vi "NotchCoeffSingleChanQTemplate.vi"(0 "notch frequency":dbl=2.0 format="%#_6p", 5 "Q factor":dbl=20.0 format="%#_6p", 9 "sample rate":dbl=50000.0 format="%#_6p", 11 "error in (no error)":errorcluster) -> (4 "scaled coefficients":i32[](array[numeric]), 15 "error out":errorcluster)   [LabVIEW 2017, in "NI_FpgaMspHost.lvlib"]
doc: "This VI designs a Butterworth filter, then quantizes and formats the coefficients into 32-bit integers for use by the Butterworth Filter VI on the FPGA.\n\nThe user is responsible for ensuring that the configuration is valid. The following restrictions apply:\nCutoff frequency must meet Nyquist criterion.\nMultichannel filters are restricted to 2nd order.\nFilter order and type cannot be changed at run-time."
uses:
  <vilib>/rvi/Analysis/host/Public/NI_FpgaMspHost.lvlib
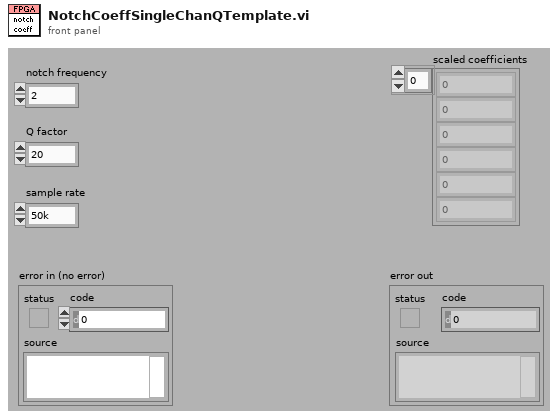
[diagram p1: front panel]
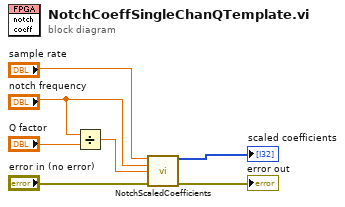
[diagram p0: block diagram]
diagram:
  n1 = Divide(x="notch frequency", y="Q factor") -> (x/y=w1:dbl)
  n2 = call <vilib>:"NotchScaledCoefficients.vi"("sample rate (S/s)"="sample rate", "notch frequency (Hz)"="notch frequency", "notch width (Hz)"=w1, "error in (no error)"="error in (no error)") -> ("scaled coefficients"=→"scaled coefficients":i32[], "error out"=→"error out":errorcluster)  [unwired: 2 in, 8 out]
